vi "CH3.vi"() -> ()   [LabVIEW 2021]
panel:
  in  "CH3":cluster{"CH3 Array":dbl[], "CH3 Message":string}
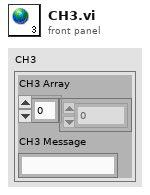
[diagram p1: front panel]
diagram:
